vi "FTW-Endpoint-TCP-Address-Decompose.vi"(0 "Endpoint Address":string, 11 "error in":errorcluster) -> (4 "Domain":string, 6 "Port":u16, 8 "Service Name":string, 15 "error out":errorcluster)   [LabVIEW 2013, in "FTW-Endpoint-TCP.lvclass"]
uses:
  FTW-Endpoint-TCP.lvclass
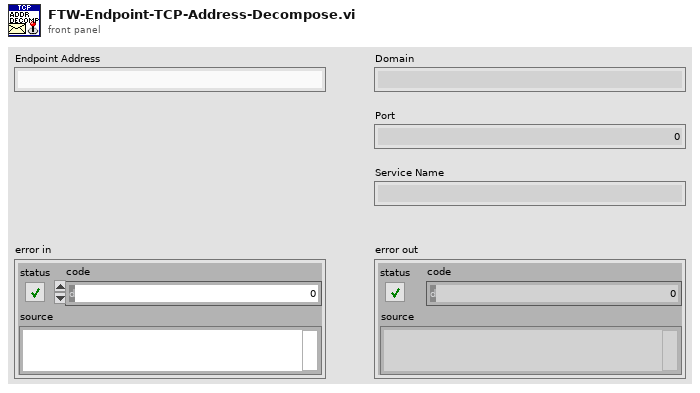
[diagram p1: front panel]
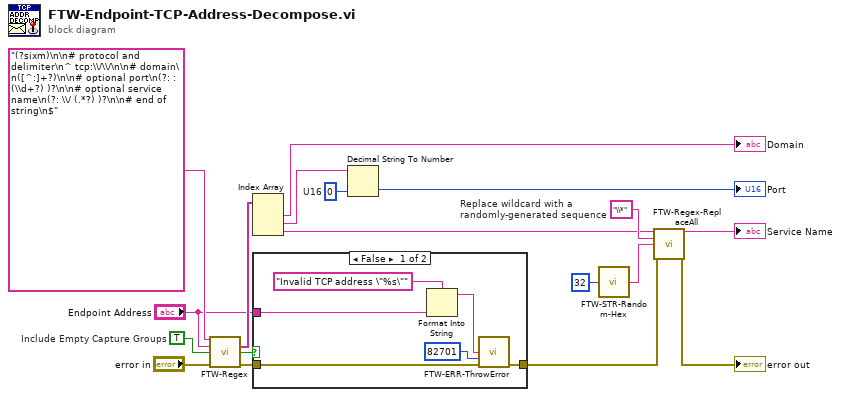
[diagram p0: block diagram]
diagram:
  w7 = "\\*"  # Replace wildcard with a randomly-generated sequence
  w8 = TRUE  # Include Empty Capture Groups
  w10 = u16 0  # U16
  n1 = call "FTW-Regex.vi"("Regular Expression"="(?sixm)\n\n# protocol and delimiter\n^ tcp:\\/\\/\n\n# domain\n([^:]+?)\n\n# optional port\n(?: : (\\d+?) )?\n\n# optional service name\n(?: \\/ (.*?) )?\n\n# end of string\n$" ("input string"), "Input String"="Endpoint Address", "Include Empty Capture Groups (F)"=w8, "error in"="error in") -> ("Submatches"=w15:string[], "Match Found?"=w14:bool, "error out"=w16:errorcluster)  [unwired: 7 in, 2 out]
  n2 = Index Array(array=w15) -> (element #1=→"Domain":string, element #2=w12:string, element #3=w4:string)  [unwired: 3 in]
  n3 = case shown="False" w14 {
    tunnel: w16 -> [w24 w25]
    tunnel: [w23 w25] -> w2
    tunnel: "Endpoint Address" -> [w19 _]
    frame False {
      n4 = Format Into String(format string="Invalid TCP address \"%s\"" ("Error Message"), w19) -> (resulting string=w20:string)  [unwired: 2 in, 1 out]
      n5 = call "FTW-ERR-ThrowError.vi"("Error Message"=w20, "Error Code"=82701, "error in"=w24) -> ("error out"=w23:errorcluster)  [unwired: 12 in]
    }
    frame True {
    }
  }
  n6 = Decimal String To Number(string=w12, default (0L)=w10) -> (number=→"Port":u16)  [unwired: 1 in, 1 out]
  n7 = call "FTW-STR-Random-Hex.vi"("String Length"=32) -> ("Random Hex String"=w5:string)  [unwired: 3 in]
  n8 = call "FTW-Regex-ReplaceAll.vi"("String"=w4, "Search for (Regular Expression)"=w7, "Replace with"=w5, "error in"=w2) -> ("String out"=→"Service Name":string, "error out"=→"error out":errorcluster)  [unwired: 9 in, 1 out]
